vi "externalDAQ.vi"(9 "customQueue":refnum<queue>, 11 "parentQueue":refnum<queue>) -> ()   [LabVIEW 2018]
uses:
  MHI Theme 6/External acquisition box/mesageHandlerTypeDef.ctl
panel:
  out "Waveform Chart":T1(graph)
  out "M dot":dbl
  out "Tin Old":dbl format="%#.2g"
  out "Tout":dbl format="%#.2g"
  out "Tin":dbl format="%#.2g"
  out "Pout":dbl format="%#_3g"
  out "Pin":dbl format="%#_3g"
  in  "offset":bool
  out "Table Control":string[][](table)
  in  "filename":string
  in  "folder":path
  in  "seconds":dbl=2.0
  in  "time limited":bool
  in  "log":bool
  in  "DAQmx Task Name":refnum<k21>="Theme6ExternalConfig5"
  in  "really stop":bool
  out "ballValve":dbl caption="ball Valve"
  out "butterflyValve":dbl caption="butterfly Valve"
  out "speed":dbl caption="compressor Speed"
  in  "quit":bool
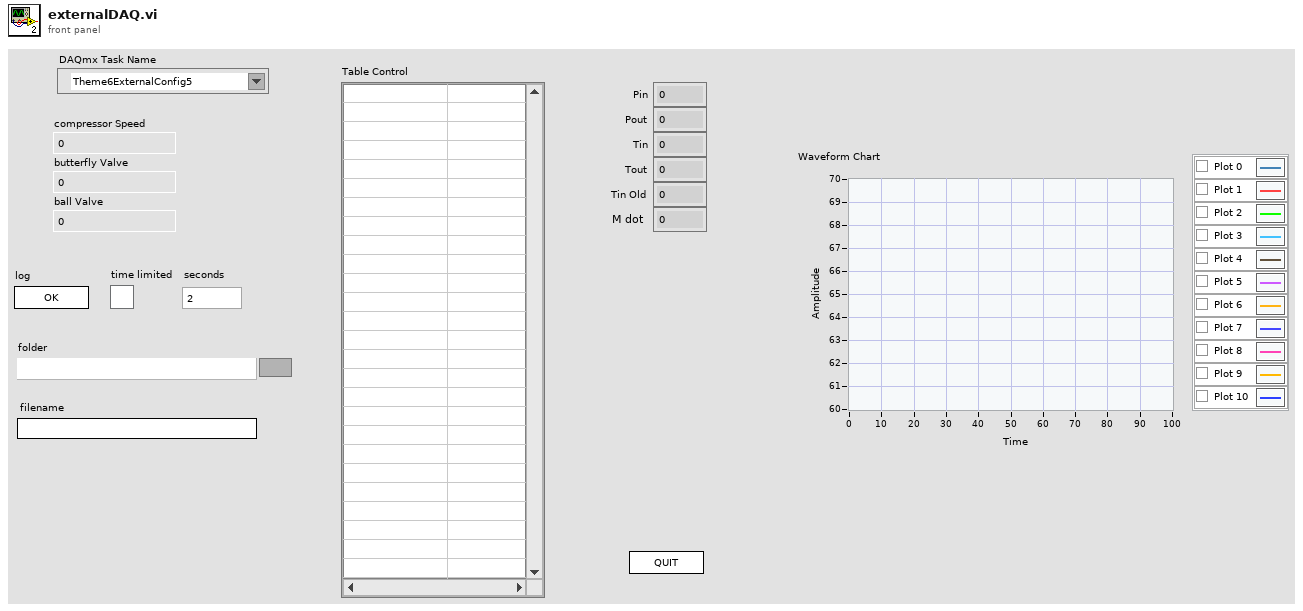
[diagram p1: front panel]
types:
  T1 = cluster{"subset[0]":dbl, "subset[1]":dbl, "subset[2]":dbl, "subset[3]":dbl, "subset[4]":dbl, "subset[5]":dbl, "subset[6]":dbl, "subset[7]":dbl, "subset[8]":dbl}
  T2 = enum8{"Enabled", "Disabled", "Disabled and Grayed Out"}
  T3 = typedef "mesageHandlerTypeDef.ctl" = cluster{"scanivalveOffset":dbl[], "scanivalvePressures":dbl[], "ambient":cluster{"Pressure":sgl, "Temperature":dbl}, "logging":bool, "displayUpdate":u16, "channels":string[], "time limited":bool, "timeLimit":dbl, "channelNames":string[], "channelUnits":string[], "rigData":dbl[], "offset":bool, "channelOffsets":dbl[]}
  T4 = cluster{"AmbientPressure(Pa)":sgl, "LabTemp":dbl}
  T5 = cluster{"[0]":dbl, "[1]":dbl, "[2]":dbl, "[3]":dbl, "[4]":dbl, "[5]":dbl, "[6]":dbl, "[7]":dbl, "[8]":dbl}
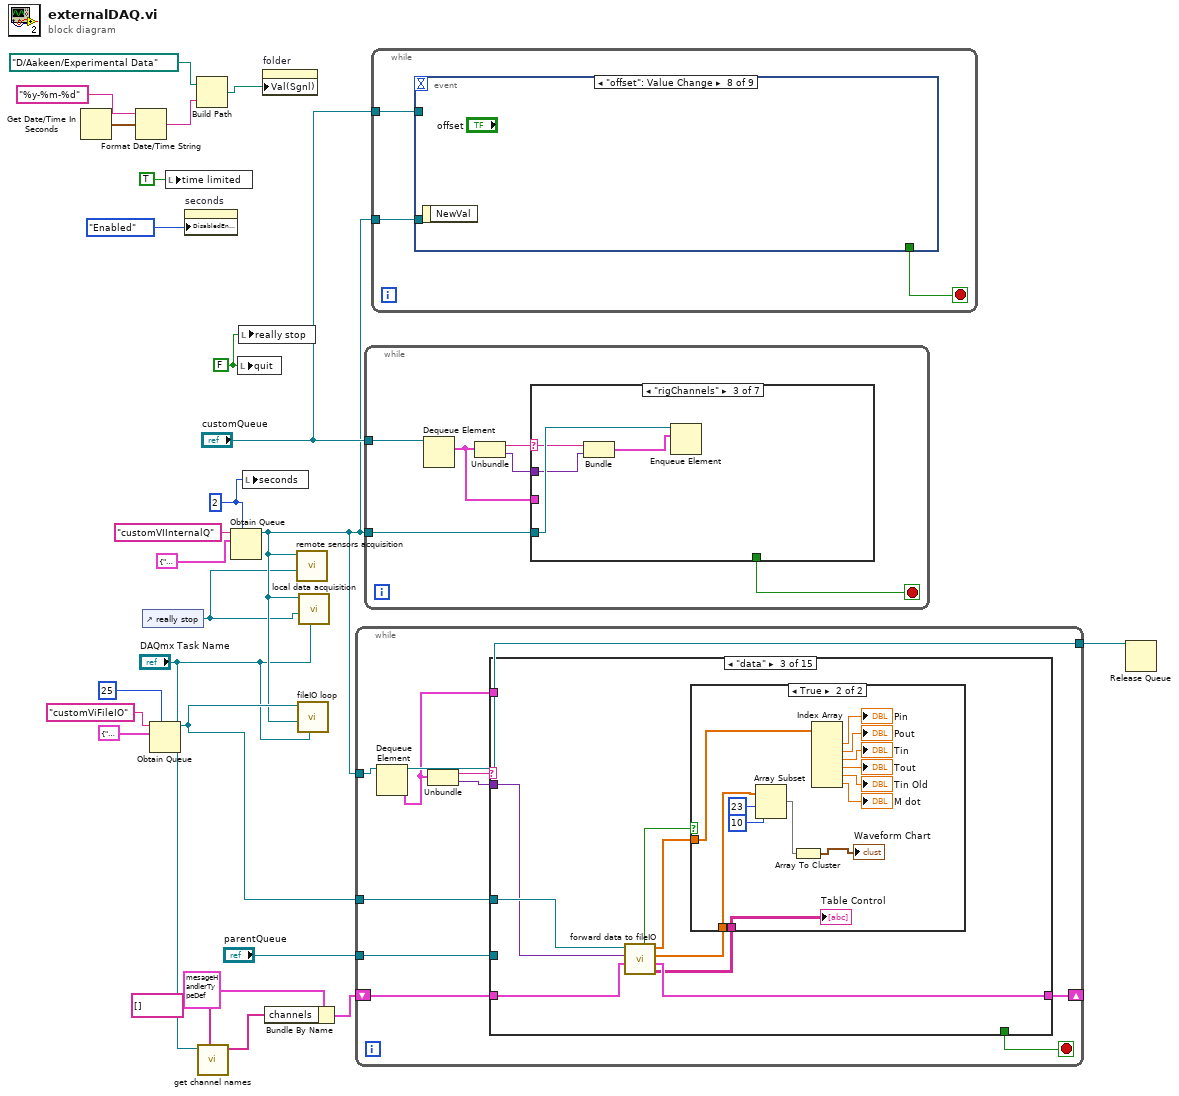
[diagram p0: block diagram]
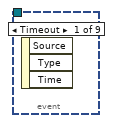
[diagram p2: hidden frame]
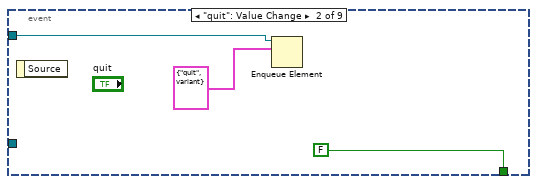
[diagram p3: hidden frame]
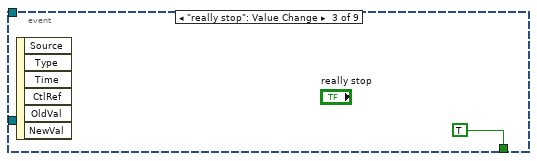
[diagram p4: hidden frame]
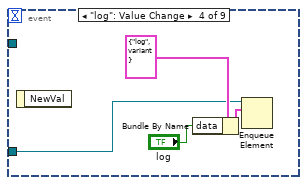
[diagram p5: hidden frame]
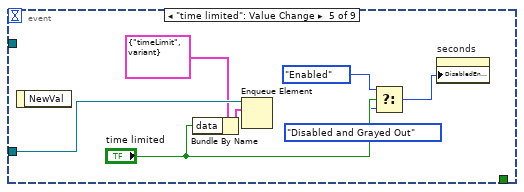
[diagram p6: hidden frame]
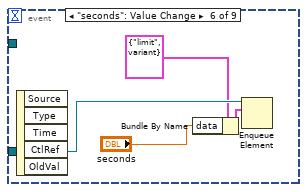
[diagram p7: hidden frame]
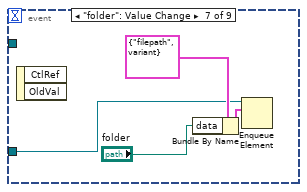
[diagram p8: hidden frame]
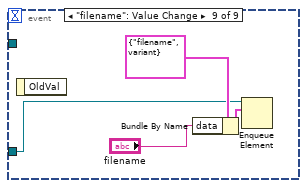
[diagram p9: hidden frame]
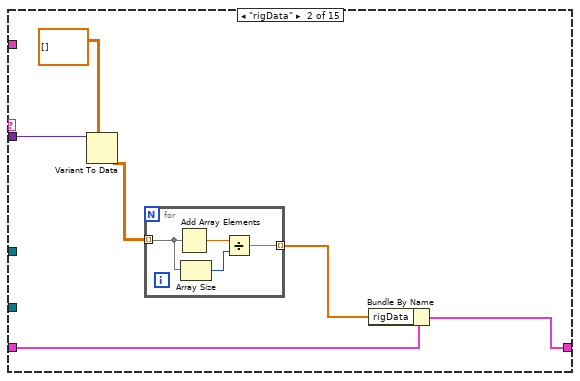
[diagram p11: hidden frame]
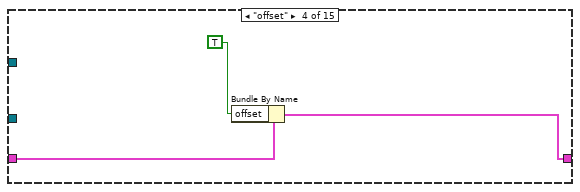
[diagram p13: hidden frame]
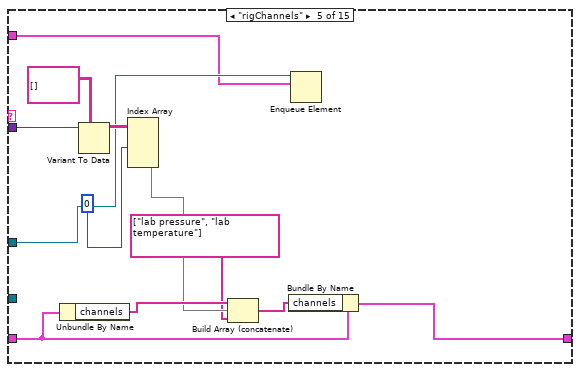
[diagram p14: hidden frame]
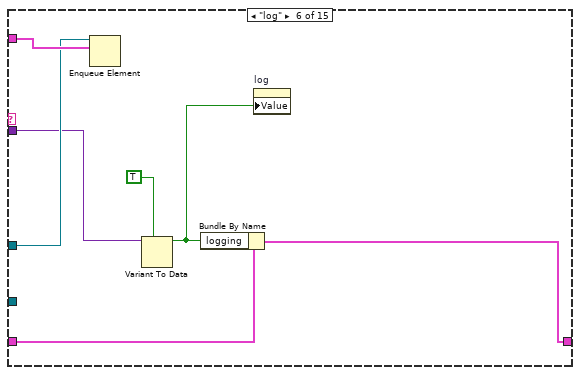
[diagram p15: hidden frame]
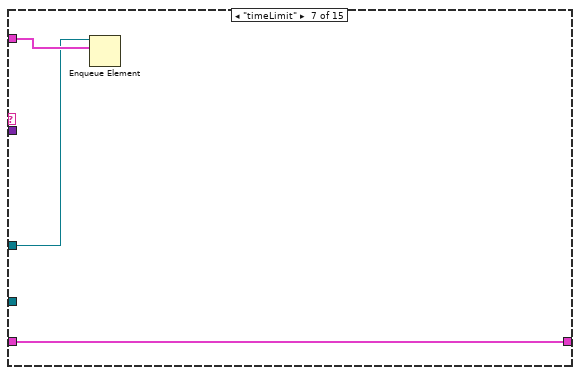
[diagram p16: hidden frame]
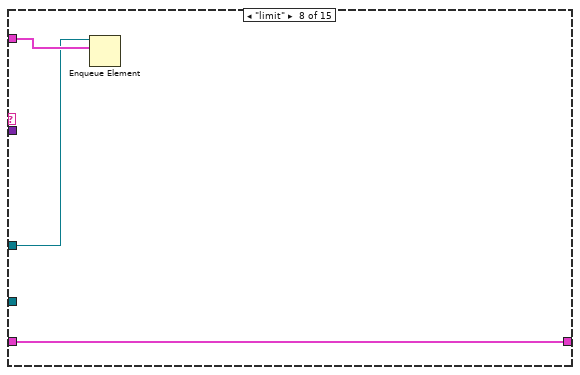
[diagram p17: hidden frame]
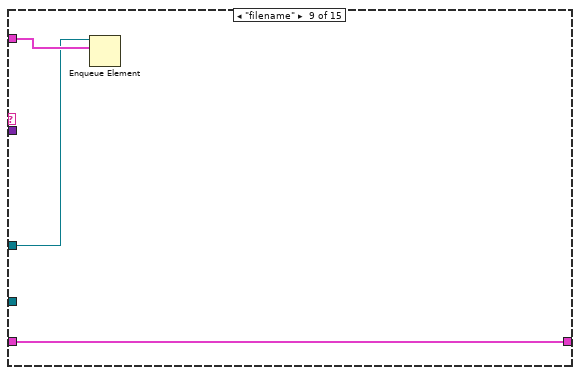
[diagram p18: hidden frame]
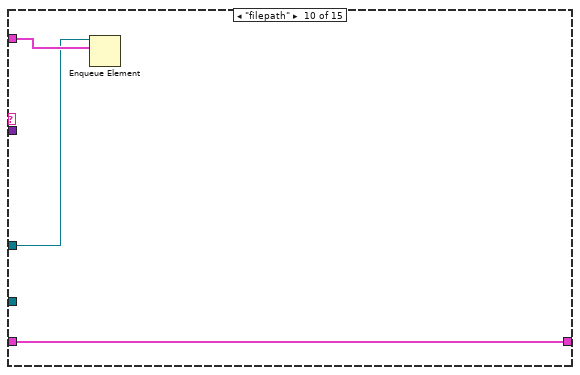
[diagram p19: hidden frame]
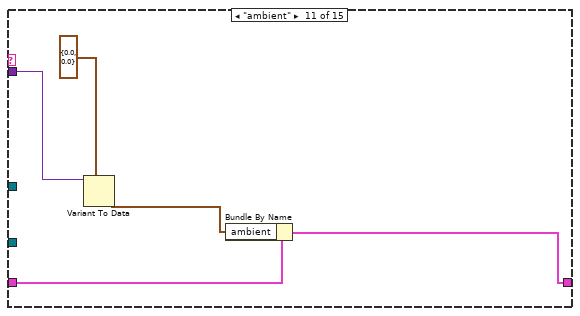
[diagram p20: hidden frame]
diagram:
  w1 = FALSE ("quit")
  w16 = 2 ("max queue size (-1, unlimited)")
  n1 = Get Date/Time In Seconds() -> (seconds since 1Jan1904=w3:timestamp)
  n2 = Format Date/Time String(time format string (%c)="%y-%m-%d", seconds (now)=w3) -> (date/time string=w4:string)  [unwired: 1 in]
  n3 = control-ref of="really stop"() -> (w12:refnum<vi>)
  n4 = Obtain Queue(max queue size (-1, unlimited)=25, name (unnamed)="customViFileIO", element data type=cluster{"message":string, "data":variant} {"message"="", "data"=variant}) -> (queue out=w17:refnum<queue>)  [unwired: 2 in, 2 out]
  n5 = local write "time limited"(TRUE) -> ()
  n6 = property on="seconds" class="DigNum (strict)"("DisabledEnum"=T2."Enabled" ("Disabled")) -> ()  [unwired: 2 in, 2 out]
  n7 = Build Path(base path=path "D:/Aakeen/Experimental Data" ("folder"), name or relative path=w4) -> (appended path=w14:path)
  n8 = call "get channel names.vi"("rigChannels"=string[] [], "DAQmx Task Name"="DAQmx Task Name") -> ("channel names"=w8:string[])  [unwired: 8 in, 1 out]
  n9 = Obtain Queue(max queue size (-1, unlimited)=w16, name (unnamed)="customVIInternalQ", element data type=cluster{"message":string, "data":variant} {"message"="", "data"=variant} ("element")) -> (queue out=w13:refnum<queue>)  [unwired: 2 in, 2 out]
  n10 = local write "quit"(w1) -> ()
  n11 = local write "really stop"(w1) -> ()
  n12 = local write "seconds"(w16) -> ()
  n13 = property on="folder" class="Path"("Val(Sgnl)"=w14) -> ()  [unwired: 2 in, 2 out]
  n14 = Bundle By Name(cluster=T3 {"scanivalveOffset"=[], "scanivalvePressures"=[], "ambient"={"Pressure"=0.0, "Temperature"=0.0}, "logging"=FALSE, "displayUpdate"=0, "channels"=[], "time limited"=FALSE, "timeLimit"=0.0, "channelNames"=[], "channelUnits"=[], "rigData"=[], "offset"=FALSE, "channelOffsets"=[]} ("Cluster in"), "channels"=w8) -> (w9:T3)
  n15 = call "remote sensors acquisition.vi"("Stop ref"=w12, "Queue in"=w13) -> ()  [unwired: 10 in]
  n16 = call "fileIO loop.vi"("DAQmx Task Name"="DAQmx Task Name", "mesageHandler in"=w13, "fileIO in"=w17) -> ()  [unwired: 9 in]
  n17 = call "local data acquisition.vi"("DAQmx Task Name"="DAQmx Task Name", "Boolean in"=w12, "message queue"=w13) -> ()  [unwired: 9 in]
  n18 = while {
    tunnel: w13 -> [w30]
    tunnel: "parentQueue" -> [w32]
    tunnel: [w30] -> w22
    shift-right: [w29] -> _
    shift-left: w9 -> [w28]
    tunnel: w17 -> [w27]
    stop <- w31 stop-if-true
    n19 = Dequeue Element(queue=w30) -> (element=w26:cluster{"message":string, "data":variant})  [unwired: 2 in, 3 out]
    n20 = Unbundle(w26) -> ("message"=w34:string, "data"=w33:variant)
    n21 = case shown="\"data\"" w34 {
      tunnel: w33 -> [_ w39 w52 _ w81 w84 _ _ _ _ w103 w108 w113 w123 _]
      tunnel: w32 -> [_ _ _ _ _ _ _ _ _ _ _ _ _ _ w133]
      tunnel: [_ _ _ _ _ _ _ _ _ _ _ _ _ _ TRUE] -> w31
      tunnel: [w35 w38 w50 w68 w75 w87 w89 w92 w95 w98 w104 w109 w114 w124 w130] -> w29
      tunnel: w28 -> [w35 w40 w51 w69 w74 w88 w89 w92 w95 w98 w105 w110 w115 w124 w130]
      tunnel: w27 -> [_ _ w53 _ w77 w85 w90 w93 w96 w99 _ _ _ _ w129]
      tunnel: w26 -> [_ _ _ _ w76 w86 w91 w94 w97 w100 _ _ _ _ _]
      frame "", Default {
      }
      frame "rigData" {
        n22 = Variant To Data(type=dbl[][] [], Variant=w39) -> (data=w37:dbl[][])  [unwired: 1 in, 1 out]
        n23 = for {
          tunnel: w37 -> [w45] mode=indexing
          tunnel: [w42] -> w36 mode=indexing
          n24 = Add Array Elements(numeric array=w45) -> (sum=w44:dbl)
          n25 = Array Size(array=w45) -> (size(s)=w43:i32)
          n26 = Divide(x=w44, y=w43) -> (x/y=w42:dbl)
        }
        n27 = Bundle By Name(cluster=w40, "rigData"=w36) -> (w38:T3)
      }
      frame "data" {
        n28 = call "forward data to fileIO.vi"("Cluster in"=w51, "data"=w52, "fileIO"=w53) -> ("table data"=w49:string[][], "data out"=w50:T3, "allData"=w46:dbl[], "subset"=w48:dbl[], "show data"=w47:bool)  [unwired: 4 in]
        n29 = case shown="True" w47 {
          tunnel: w49 -> [_ w66]
          tunnel: w48 -> [_ w58]
          tunnel: w46 -> [_ w54]
          frame False {
          }
          frame True {
            n30 = Array Subset(array=w54, index=23, length=10) -> (w56:dbl[])
            n31 = Array To Cluster(array=w56) -> (cluster=→"Waveform Chart":T5)
            n32 = Index Array(array=w58) -> (element #1=→"Pin":dbl, element #2=→"Pout":dbl, element #3=→"Tin":dbl, element #4=→"Tout":dbl, element #5=→"Tin Old":dbl, element #6=→"M dot":dbl)  [unwired: 6 in]
            "Table Control" <- w66
          }
        }
      }
      frame "offset" {
        n33 = Bundle By Name(cluster=w69, "offset"=TRUE) -> (w68:T3)
      }
      frame "rigChannels" {
        n34 = Unbundle By Name(w74) -> ("channels"=w73:string[])
        n35 = Variant To Data(type=string[][] [], Variant=w81) -> (data=w79:string[][])  [unwired: 1 in, 1 out]
        n36 = Index Array(array=w79, index (col) #1=0 ("index (row)")) -> (element #1=w71:string[])  [unwired: 3 in, 1 out]
        n37 = Build Array (concatenate)(w73, w71, string[] ["lab pressure", "lab temperature"] ("delimiter (Tab)")) -> (w72:string[])
        n38 = Bundle By Name(cluster=w74, "channels"=w72) -> (w75:T3)
        n39 = Enqueue Element(queue=w77, element=w76) -> ()  [unwired: 2 in, 3 out]
      }
      frame "log" {
        n40 = Enqueue Element(queue=w85, element=w86) -> ()  [unwired: 2 in, 3 out]
        n41 = Variant To Data(type=TRUE, Variant=w84) -> (data=w82:bool)  [unwired: 1 in, 1 out]
        n42 = Bundle By Name(cluster=w88, "logging"=w82) -> (w87:T3)
        n43 = property on="log" class="Bool (strict)"("Value"=w82) -> ()  [unwired: 2 in, 2 out]
      }
      frame "timeLimit" {
        n44 = Enqueue Element(queue=w90, element=w91) -> ()  [unwired: 2 in, 3 out]
      }
      frame "limit" {
        n45 = Enqueue Element(queue=w93, element=w94) -> ()  [unwired: 2 in, 3 out]
      }
      frame "filename" {
        n46 = Enqueue Element(queue=w96, element=w97) -> ()  [unwired: 2 in, 3 out]
      }
      frame "filepath" {
        n47 = Enqueue Element(queue=w99, element=w100) -> ()  [unwired: 2 in, 3 out]
      }
      frame "ambient" {
        n48 = Variant To Data(type=T4 {"AmbientPressure(Pa)"=0.0, "LabTemp"=0.0} ("output cluster"), Variant=w103) -> (data=w101:T4)  [unwired: 1 in, 1 out]
        n49 = Bundle By Name(cluster=w105, "ambient"=w101) -> (w104:T3)
      }
      frame "scanivalve" {
        n50 = Variant To Data(type=dbl[] [] ("y"), Variant=w108) -> (data=w106:dbl[])  [unwired: 1 in, 1 out]
        n51 = Bundle By Name(cluster=w110, "scanivalvePressures"=w106) -> (w109:T3)
      }
      frame "scanivalveZero" {
        n52 = Variant To Data(type=dbl[] [] ("y"), Variant=w113) -> (data=w111:dbl[])  [unwired: 1 in, 1 out]
        n53 = Bundle By Name(cluster=w115, "scanivalveOffset"=w111) -> (w114:T3)
      }
      frame "filenameUpdate" {
        n54 = Variant To Data(type=dbl[] [] ("y"), Variant=w123) -> (data=w121:dbl[])  [unwired: 1 in, 1 out]
        n55 = for {
          tunnel: w121 -> [w127] mode=indexing
          tunnel: [w125] -> w120 mode=indexing
          n56 = Format Value(format string="%d", value (0)=w127) -> (output string=w125:string)  [unwired: 1 in]
        }
        n57 = Index Array(array=w120) -> (element #1=w119:string, element #2=w118:string)  [unwired: 2 in]
        n58 = Concatenate Strings(w119, "kRPM - ", w118) -> (w116:string)
        n59 = property on="filename" class="Str"("Val(Sgnl)"=w116) -> ()  [unwired: 2 in, 2 out]
      }
      frame "quit" {
        n60 = Enqueue Element(queue=w133, element=cluster{"message":string, "data":variant} {"message"="customVIQuit", "data"=variant}) -> ()  [unwired: 2 in, 3 out]
        n61 = Enqueue Element(queue=w129, element=cluster{"message":string, "data":variant} {"message"="quit", "data"=variant}) -> ()  [unwired: 2 in, 3 out]
      }
    }
  }
  n62 = while {
    tunnel: "customQueue" -> [w139]
    tunnel: w13 -> [w136]
    stop <- w135 stop-if-true
    n63 = Dequeue Element(queue=w139) -> (element=w134:cluster{"message":string, "data":variant})  [unwired: 2 in, 3 out]
    n64 = Unbundle(w134) -> ("message"=w138:string, "data"=w137:variant)
    n65 = case shown="\"rigChannels\"" w138 {
      selector: w138 -> [_ _ w144 _ _ _ _]
      tunnel: w137 -> [_ w142 w146 w155 w163 w166 _]
      tunnel: w136 -> [_ w143 w147 w153 w157 _ w169]
      tunnel: [_ _ _ _ _ _ TRUE] -> w135
      tunnel: w134 -> [_ _ _ _ _ _ _]
      frame "False", Default {
      }
      frame "data" {
        n66 = Bundle("rigData", "data"=w142) -> (w141:cluster{string, "data":variant})  [unwired: 1 in]
        n67 = Enqueue Element(queue=w143, element=w141) -> ()  [unwired: 2 in, 3 out]
      }
      frame "rigChannels" {
        n68 = Bundle(w144, "data"=w146) -> (w145:cluster{string, "data":variant})  [unwired: 1 in]
        n69 = Enqueue Element(queue=w147, element=w145) -> ()  [unwired: 2 in, 3 out]
      }
      frame "speedChange" {
        n70 = local read "butterflyValve"() -> (w151:dbl)
        n71 = Variant To Data(type=0.0 ("y"), Variant=w155) -> (data=w152:dbl)  [unwired: 1 in, 1 out]
        "speed" <- w152
        n72 = Build Array(w152, w151) -> (w148:dbl[])
        n73 = Bundle By Name(cluster=cluster{"message":string, "data":variant} {"message"="filenameUpdate", "data"=variant} ("element"), "data"=w148) -> (w149:cluster{"message":string, "data":variant})
        n74 = Enqueue Element(queue=w153, element=w149) -> ()  [unwired: 2 in, 3 out]
      }
      frame "butterflyChange" {
        n75 = Variant To Data(type=0.0 ("y"), Variant=w163) -> (data=w158:dbl)  [unwired: 1 in, 1 out]
        "butterflyValve" <- w158
        n76 = local read "speed"() -> (w156:dbl)
        n77 = Build Array(w156, w158) -> (w161:dbl[])
        n78 = Bundle By Name(cluster=cluster{"message":string, "data":variant} {"message"="filenameUpdate", "data"=variant} ("element"), "data"=w161) -> (w160:cluster{"message":string, "data":variant})
        n79 = Enqueue Element(queue=w157, element=w160) -> ()  [unwired: 2 in, 3 out]
      }
      frame "ballChange" {
        n80 = Variant To Data(type=0.0 ("y"), Variant=w166) -> (data=→"ballValve":dbl)  [unwired: 1 in, 1 out]
      }
      frame "quit" {
        n81 = property on="really stop" class="Bool (strict)"("Val(Sgnl)"=TRUE) -> ()  [unwired: 2 in, 2 out]
        n82 = Enqueue Element(queue=w169, element=cluster{"message":string, "data":variant} {"message"="quit", "data"=variant}) -> ()  [unwired: 2 in, 3 out]
      }
    }
  }
  n83 = while {
    tunnel: w13 -> [w173]
    tunnel: "customQueue" -> [w171]
    stop <- w172 stop-if-true
    n84 = event shown="[7] \"offset\": Value Change" {
      selector: _ -> [_ _ _ _ _ _ _ _ _]
      dyn-events: _ -> [_ _ _ _ _ _ _ _ _]
      timeout: _ -> [_ _ _ _ _ _ _ _ _]
      tunnel: w173 -> [_ _ _ w178 w188 w192 w193 _ w197]
      tunnel: [_ FALSE TRUE _ _ _ _ _ _] -> w172
      tunnel: w171 -> [_ w174 _ _ _ _ _ _ _]
      event Timeout {
        n85 = event-data() -> ()  [unwired: 1 in, 3 out]
      }
      event "quit": Value Change {
        n86 = event-data() -> ()  [unwired: 1 in, 1 out]
        n87 = Enqueue Element(queue=w174, element=cluster{"message":string, "data":variant} {"message"="quit", "data"=variant}) -> ()  [unwired: 2 in, 3 out]
      }
      event "really stop": Value Change {
        n88 = event-data() -> ()  [unwired: 1 in, 6 out]
      }
      event "log": Value Change {
        n89 = event-data() -> ()  [unwired: 1 in, 1 out]
        n90 = Bundle By Name(cluster=cluster{"message":string, "data":variant} {"message"="log", "data"=variant} ("element"), "data"="log") -> (w180:cluster{"message":string, "data":variant})
        n91 = Enqueue Element(queue=w178, element=w180) -> ()  [unwired: 2 in, 3 out]
      }
      event "time limited": Value Change {
        n92 = event-data() -> ()  [unwired: 1 in, 1 out]
        n93 = Bundle By Name(cluster=cluster{"message":string, "data":variant} {"message"="timeLimit", "data"=variant} ("element"), "data"="time limited") -> (w186:cluster{"message":string, "data":variant})
        n94 = Enqueue Element(queue=w188, element=w186) -> ()  [unwired: 2 in, 3 out]
        n95 = Select(t=T2."Enabled" ("Disabled"), s="time limited", f=T2."Disabled and Grayed Out" ("Disabled")) -> (s? t:f=w182:T2)
        n96 = property on="seconds" class="DigNum (strict)"("DisabledEnum"=w182) -> ()  [unwired: 2 in, 2 out]
      }
      event "seconds": Value Change {
        n97 = event-data() -> ()  [unwired: 1 in, 5 out]
        n98 = Bundle By Name(cluster=cluster{"message":string, "data":variant} {"message"="limit", "data"=variant} ("element"), "data"="seconds") -> (w190:cluster{"message":string, "data":variant})
        n99 = Enqueue Element(queue=w192, element=w190) -> ()  [unwired: 2 in, 3 out]
      }
      event "folder": Value Change {
        n100 = event-data() -> ()  [unwired: 1 in, 2 out]
        n101 = Bundle By Name(cluster=cluster{"message":string, "data":variant} {"message"="filepath", "data"=variant} ("element"), "data"="folder") -> (w195:cluster{"message":string, "data":variant})
        n102 = Enqueue Element(queue=w193, element=w195) -> ()  [unwired: 2 in, 3 out]
      }
      event "offset": Value Change {
        n103 = event-data() -> ()  [unwired: 1 in, 1 out]
      }
      event "filename": Value Change {
        n104 = event-data() -> ()  [unwired: 1 in, 1 out]
        n105 = Bundle By Name(cluster=cluster{"message":string, "data":variant} {"message"="filename", "data"=variant} ("element"), "data"="filename") -> (w199:cluster{"message":string, "data":variant})
        n106 = Enqueue Element(queue=w197, element=w199) -> ()  [unwired: 2 in, 3 out]
      }
    }
  }
  n107 = Release Queue(queue=w22) -> ()  [unwired: 2 in, 3 out]
